vi "Const Rate Fitter.vi"() -> ()   [LabVIEW 2014]
uses:
  <vilib>/gmath/SpecialFunctions.llb/Factorial.vi
  <vilib>/Utility/file.llb/Read From Spreadsheet File (DBL).vi
  <vilib>/imath/engines/lvmath2/RunTimeEngine/BuiltInFunctions/mean/NIMS_RRow=mean(RM,I32).vi
  <vilib>/imath/engines/lvmath2/RunTimeEngine/RangeToken/NIMS_Range_R2 - Integer.vi
  <instcachedir>/0/NIMS_Range_R2 - Integer_2D1304BAF97744E0A293025746CBADFC.lvgen/NIMS_Range_R2 - Integer_2D1304BAF97744E0A293025746CBADFC_000.vi
  <vilib>/imath/engines/lvmath2/RunTimeEngine/CommandStatement/MC_CommandStatement_break.vi
  <vilib>/imath/engines/lvmath2/RunTimeEngine/IndexRead/NIMS V(S).vi
  <instcachedir>/0/NIMS V(S)_0488751826AF41519A22953C041130DC.lvgen/NIMS V(S)_0488751826AF41519A22953C041130DC_002.vi
  <vilib>/imath/engines/lvmath2/RunTimeEngine/ArithmeticOperatorToken/NIMS_ArithmeticOperator_times.vi
  <instcachedir>/0/NIMS_ArithmeticOperator_times_2EFF5B13FCA4492A81D59089AD809F54.lvgen/NIMS_ArithmeticOperator_times_2EFF5B13FCA4492A81D59089AD809F54_000.vi
  <vilib>/imath/engines/lvmath2/RunTimeEngine/IndexReplace/NIMS V(S)=V.vi
  <instcachedir>/0/NIMS V(S)=V_21D22CAE002F40F09B1F0AFCB929580F.lvgen/NIMS V(S)=V_21D22CAE002F40F09B1F0AFCB929580F_000.vi
  <vilib>/imath/engines/lvmath2/RunTimeEngine/ErrorHandling/NIMS_Create Error From Enums.vi
  <vilib>/imath/engines/lvmath2/RunTimeEngine/NodeEndStatement/NIMS_NodeEndStatement_Output.vi
  <instcachedir>/0/NIMS_NodeEndStatement_Output_53EC0D466D134D7ABD903AC30B43404B.lvgen/NIMS_NodeEndStatement_Output_53EC0D466D134D7ABD903AC30B43404B_004.vi
  <instcachedir>/0/NIMS_NodeEndStatement_Output_53EC0D466D134D7ABD903AC30B43404B.lvgen/NIMS_NodeEndStatement_Output_53EC0D466D134D7ABD903AC30B43404B_005.vi
  <vilib>/imath/engines/lvmath2/RunTimeEngine/ErrorHandling/NIMS_Finalize Error.vi
  <vilib>/Analysis/NI_AALBase.lvlib
  <vilib>/gmath/NI_Gmath.lvlib
panel:
  out "pArray":dbl[](array[numeric])
  out "Histogram Graph":cluster{"X Values":dbl[], dbl[]}[](graph)
  in  "file path (dialog if empty)":path=path "C:/Users/zchmlk/Desktop/week8-master/Const2.txt"
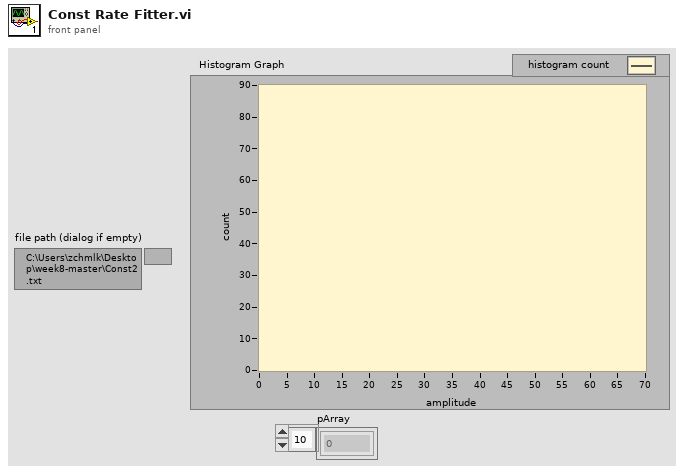
[diagram p1: front panel]
types:
  T1 = cluster{"X Values":dbl[], "Histogram: h(x)":i32[]}
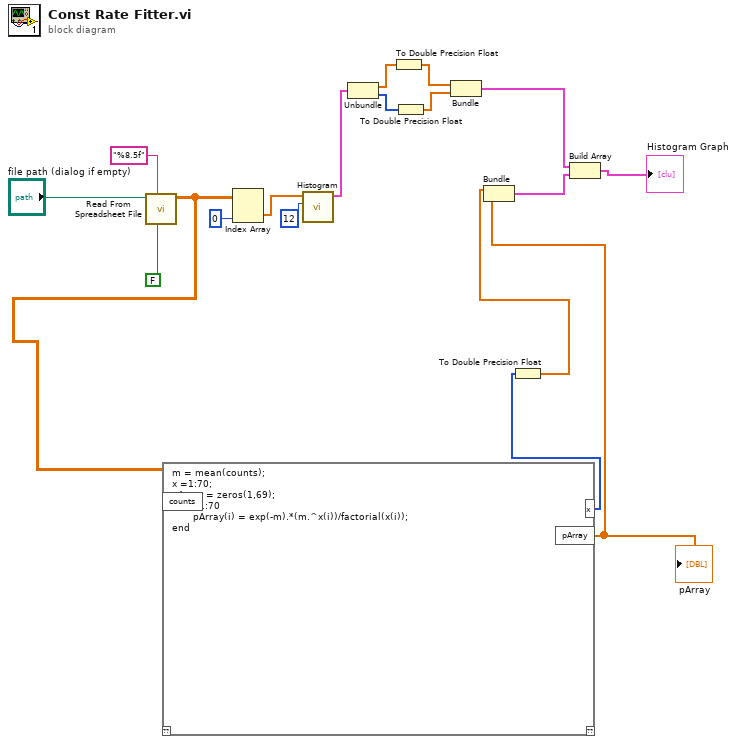
[diagram p0: block diagram]
diagram:
  n1 = call-poly <vilib>:"Read From Spreadsheet File.vi"("transpose (no:F)"=FALSE, "format (%.3f)"="%8.5f", "file path (dialog if empty)"="file path (dialog if empty)") -> ("all rows"=w4:dbl[][])  [unwired: 4 in, 4 out]
  n2 = mathscript code="m = mean(counts);\nx =1:70;\npArray = zeros(1,69);\nfor i=1:70\n       pArray(i) = exp(-m).*(m.^x(i))/factorial(x(i));       \nend"("counts"=w4) -> ("pArray"=w1:dbl[], "x"=w3:i32[])  [unwired: 1 in, 1 out]
  "pArray" <- w1
  n3 = Index Array(array=w4, index (col)=0) -> (element=w14:dbl[])  [unwired: 1 in]
  n4 = call <vilib>:"Histogram.vi"("intervals"=12, "X"=w14) -> ("Histogram Graph"=w11:T1)  [unwired: 6 in, 3 out]
  n5 = Unbundle(w11) -> ("X Values"=w6:dbl[], "Histogram: h(x)"=w10:i32[])
  n6 = To Double Precision Float(number=w6) -> (double precision float=w5:dbl[])
  n7 = To Double Precision Float(number=w10) -> (double precision float=w9:dbl[])
  n8 = Bundle(w5, w9) -> (w8:cluster{dbl[], dbl[]})  [unwired: 1 in]
  n9 = To Double Precision Float(number=w3) -> (double precision float=w7:dbl[])
  n10 = Bundle(w7, "pArray"=w1) -> (w2:cluster{dbl[], "pArray":dbl[]})  [unwired: 1 in]
  n11 = Build Array(w8, w2) -> (→"Histogram Graph":cluster{dbl[], "pArray":dbl[]}[])
